vi "ble_read_write_characteristics.vi"() -> ()   [LabVIEW 2021]
uses:
  <vilib>/BLE/type_def/connection_status_bundle.ctl
  <vilib>/BLE/type_def/address_type.ctl
  <vilib>/BLE/ble_functions/ble_write_by_service_characteristic_uint8array.vi
  <vilib>/Utility/inputDevices.llb/mouseAcquire.vi
  <vilib>/Utility/inputDevices.llb/closeMouse.vi
panel:
  in  "Emergency Stop":bool
  out "Current Mouse Coordinates":T1
  out "Mouse Status":cluster{"Clicked?":bool}
  out "Drawing":cluster{i32[], i32[]}[](graph)
  in  "Clear Drawing":bool
  out "Connected":bool
  out "Device Name":string
  in  "Address Type":T2=1 items=["Public", "Random"]
  out "Handle table":string[][](array[string])
  out "Connection Status":T3={"MAC Address"="", "cnx handle"=0, "cnx flags"=0, "Address Type"=125, "Connection Interval (ms)"=125, "Timeout(ms)"=125, "Latency"=0, "bonding handle"=0} {"Address Type" items=["Public", "Random"]}
  out "Scanning":bool
  in  "Continue":bool
  in  "MAC Address":string
  in  "COM Bluegiga in":refnum<visa-resource-name>="COM5"
  out "Devices":string[][](array[string])
  out "BLED112 Dongle Info":string
  # "This VI an example of scanning for BLE devices using the \nBLED112 Bluetooth Smart Dongle by Bluegiga\nhttps://www.bluegiga.com/en-US/products/bled112-bluetooth-smart-dongle/\n\nand\nBLE (Bluetooth Low Energy) toolkit for LabVIEW\nww.\n\nInstructions:\nBefore running the VI\n1. Select the COM port for the BLED112 USB receiver\n(You can verify this in the Device Manager)\n\n2. Run the VI\n\n3. The VI will reset the dongle and scan for available BLE devices\n \n4. Introduce the MAC Address and Address Type of the device you want to connect and click in the CONTINUE button to connect with it\n\n5. The VI will read the Characteristic 0x2A00 of the Service 0x1800 which contains \nthe Device Name\n\nhttps://www.bluetooth.com/specifications/gatt/viewer?attributeXmlFile=org.bluetooth.service.generic_access.xml&u=org.bluetooth.service.generic_access.xml"
  # "SCAN"
  # "RSSI (power)"
  # "Advertising Package Type"
  # "MAC Address"
  # "Address Type"
  # "Friendly name"
  # "DEVICES FOUND"
  # "Introduce the MAC Address and Address Type of the device you want to connect and click in the CONTINUE button"
  # "CONNECT"
  # "READING DEVICE NAME"
  # "Service 0x1800\nCharacteristic 0x2A00\nDevice Name"
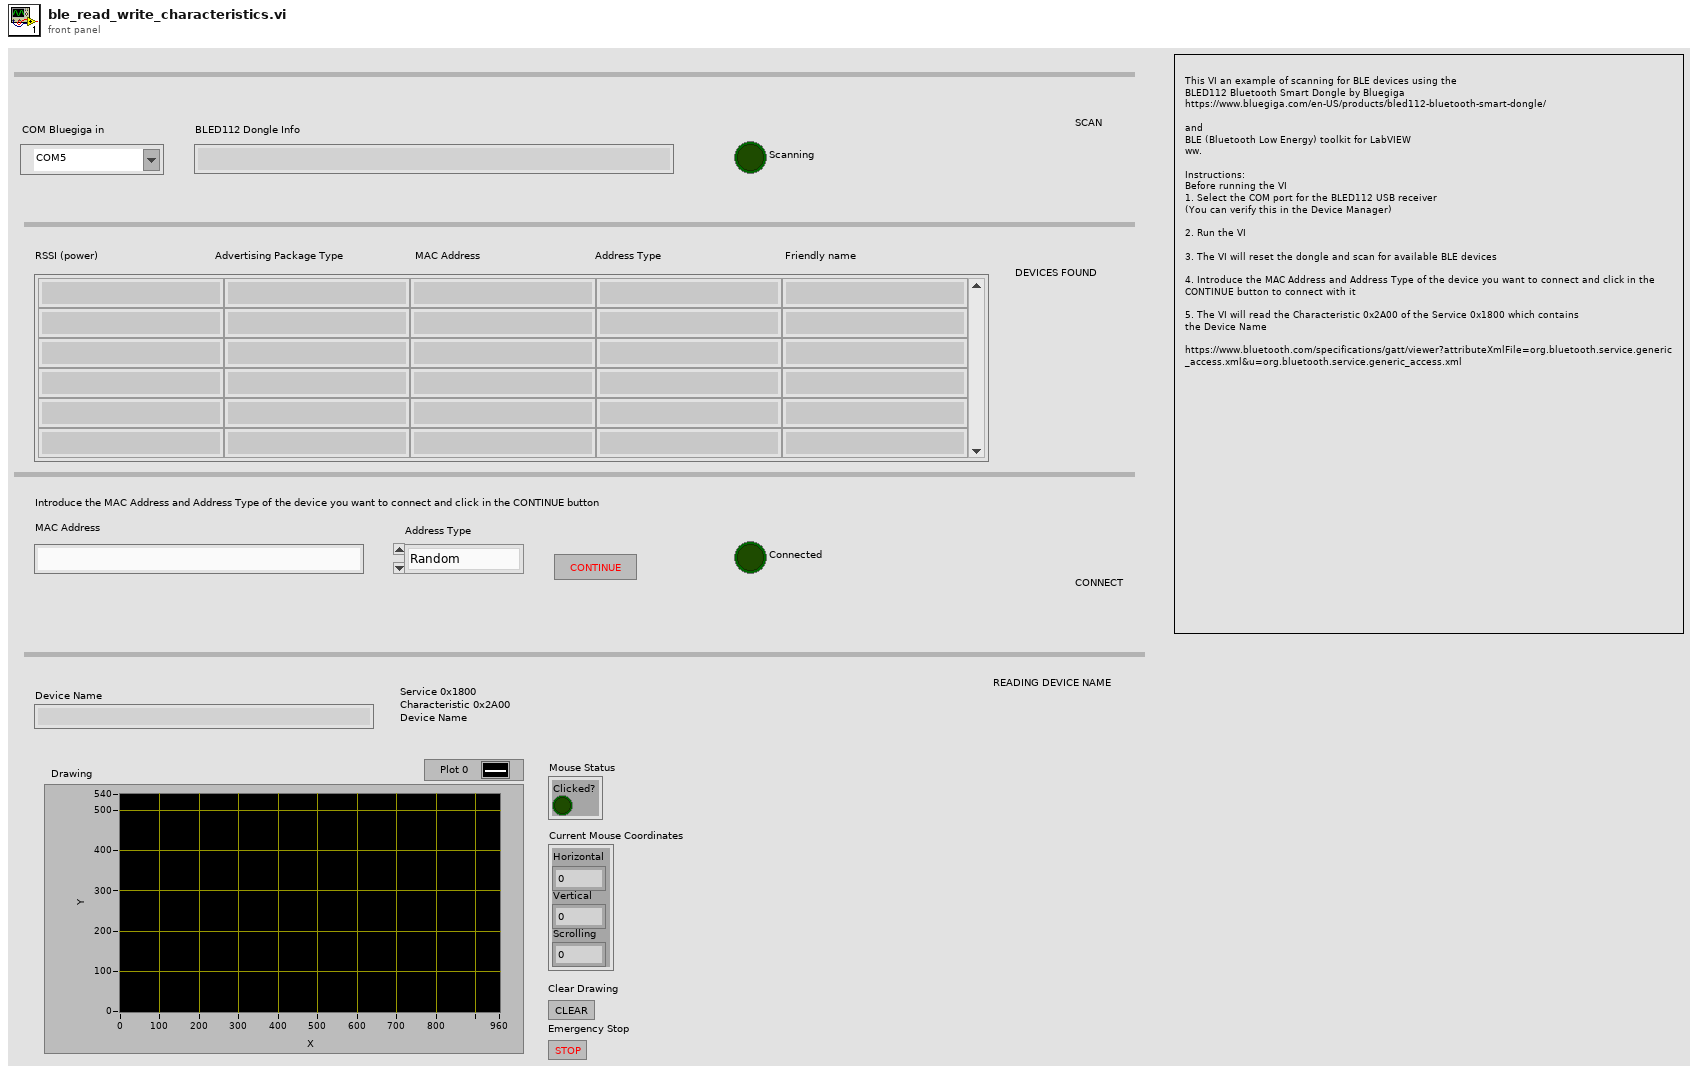
[diagram p1: front panel]
types:
  T1 = cluster{"Horizontal":i32, "Vertical":i32, "Scrolling":i32}
  T2 = typedef "address_type.ctl" = u8
  T3 = typedef "connection_status_bundle.ctl" = cluster{"MAC Address":string, "cnx handle":u8, "cnx flags":u8, "Address Type":T2, "Connection Interval (ms)":u16, "Timeout(ms)":u16, "Latency":u16, "bonding handle":u8}
  T4 = cluster{"Horizontal Array":i32[], "Vertical Array":i32[]}
  T5 = cluster{"Horizontal Array":i32[], "Vertical Array":i32[]}[]
  T6 = cluster{"button 1":bool, "button 2":bool, "button 3":bool, "button 4":bool}
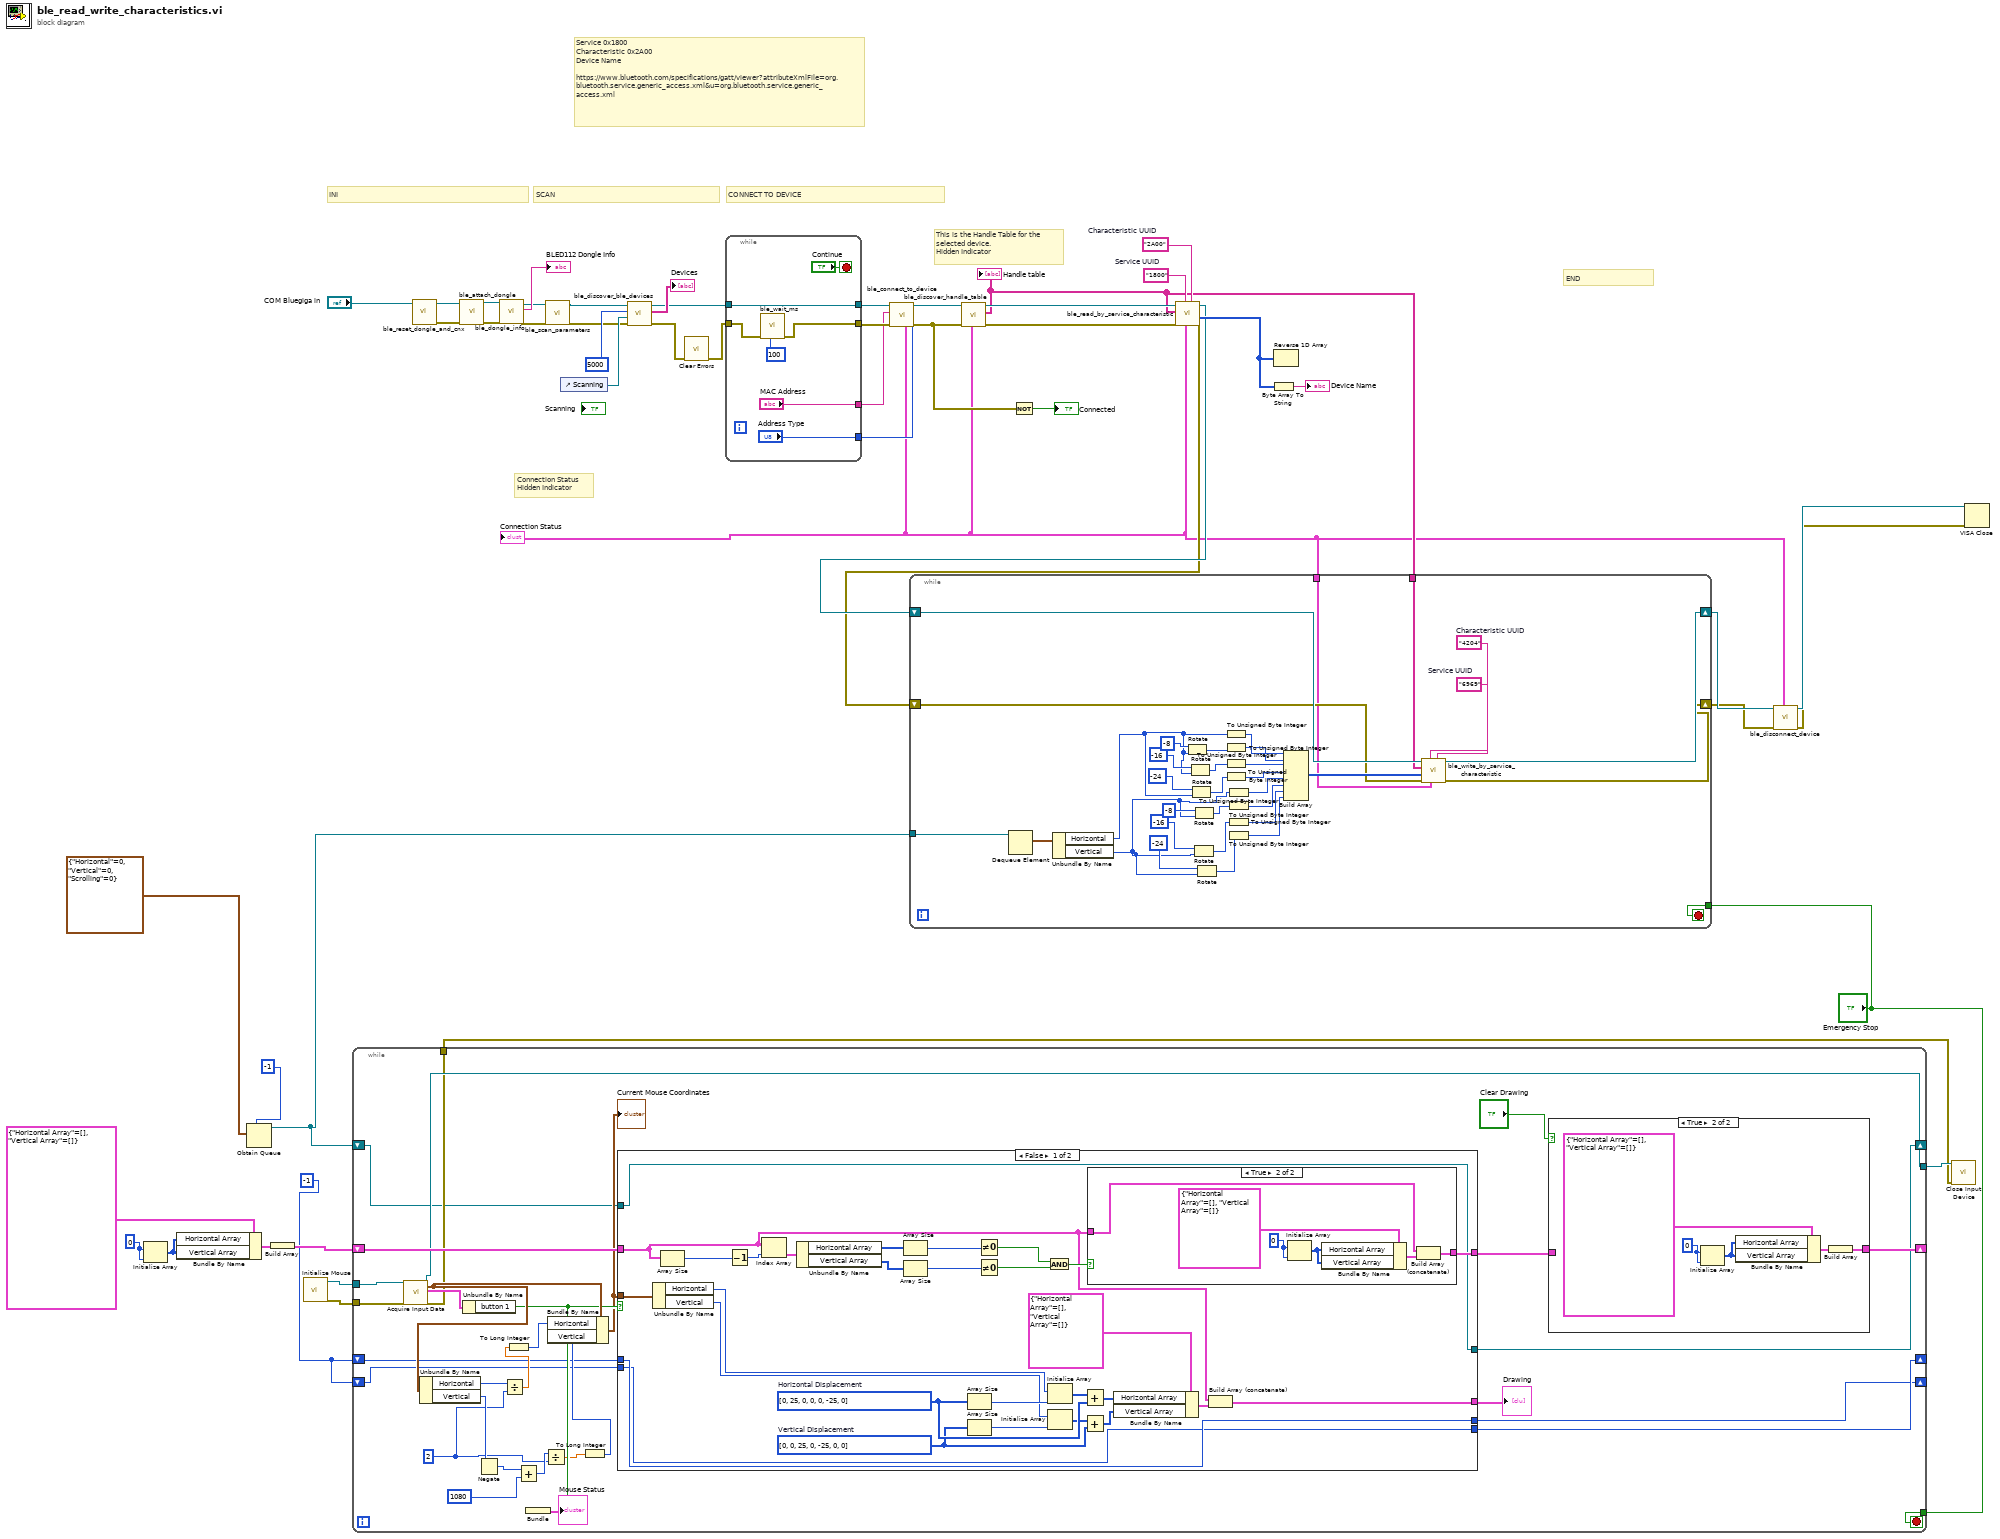
[diagram p0: block diagram]
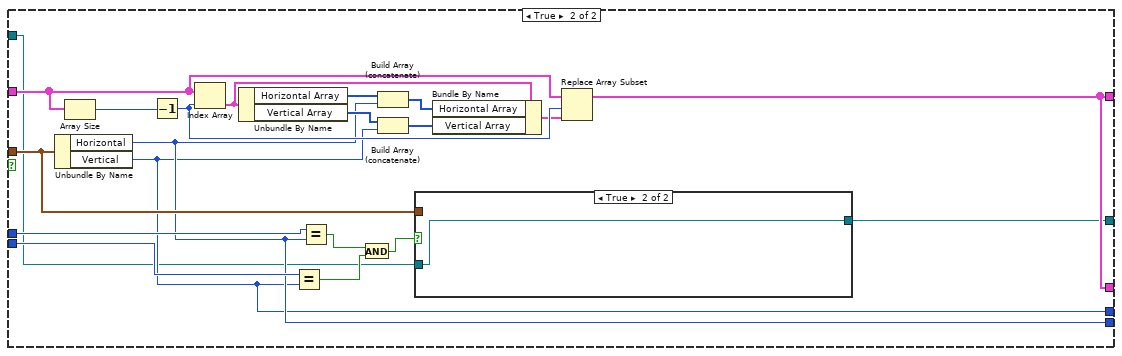
[diagram p4: hidden frame]
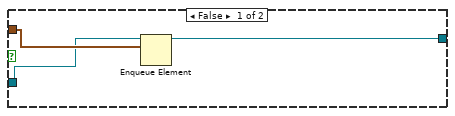
[diagram p5: hidden frame]
diagram:
  w10 = -1
  w16 = 0
  w21 = "2A00"  # Characteristic UUID
  w23 = "1800"  # Service UUID
  # "Connection Status\nHidden Indicator"
  # "Service 0x1800\nCharacteristic 0x2A00\nDevice Name\n\nhttps://www.bluetooth.com/specifications/gatt/viewer?attributeXmlFile=org.bluetooth.service.generic_access.xml&u=org.bluetooth.service.generic_access.xml"
  # "This is the Handle Table for the\nselected device. \nHidden Indicator"
  # "CONNECT TO DEVICE"
  # "SCAN"
  # "END"
  # "INI"
  n1 = Initialize Array(w16, w16) -> (w14:i32[])
  n2 = Bundle By Name(cluster=T4 {"Horizontal Array"=[], "Vertical Array"=[]}, "Horizontal Array"=w14, "Vertical Array"=w14) -> (w17:T4)
  n3 = Obtain Queue(max queue size (-1, unlimited)=-1, element data type=T1 {"Horizontal"=0, "Vertical"=0, "Scrolling"=0}) -> (queue out=w8:refnum<queue>)  [unwired: 3 in, 2 out]
  n4 = Build Array(w17) -> (w15:T5)
  n5 = call <vilib>:"Initialize Mouse.vi"() -> ("error out"=w19:errorcluster, "device ID"=w20:refnum<k1>)  [unwired: 10 in]
  n6 = while {
    tunnel: w20 -> [w82]
    tunnel: w19 -> [w81]
    shift-right: [w71] -> _
    shift-left: w15 -> [w75]
    tunnel: [w70] -> w13
    tunnel: [w69] -> w12
    shift-right: [w56] -> _
    shift-left: w10 -> [w59]
    shift-right: [w55] -> _
    shift-left: w10 -> [w58]
    shift-right: [w53] -> _
    shift-left: w8 -> [w54]
    tunnel: "Emergency Stop" -> [w52]
    stop <- w52 stop-if-true
    w62 = 2
    n7 = call-poly <vilib>:"Acquire Input Data.vi"("device ID"=w82, "error in (no error)"=w81) -> ("device ID"=w70:refnum<k1>, "axis info"=w79:T1, "button info"=w80:T6, "error out"=w69:errorcluster)  [unwired: 14 in]
    n8 = Unbundle By Name(w79) -> ("Horizontal"=w63:i32, "Vertical"=w78:i32)
    n9 = Unbundle By Name(w80) -> ("button 1"=w76:bool)
    n10 = Negate(x=w78) -> (-x=w68:i32)
    n11 = Divide(x=w63, y=w62) -> (x/y=w60:dbl)
    n12 = To Long Integer(number=w60) -> (32bit integer=w61:i32)
    n13 = Add(x=w68, y=1080) -> (x+y=w66:i32)
    n14 = Bundle("button 1"=w76) -> (→"Mouse Status":cluster{"button 1":bool})  [unwired: 1 in]
    n15 = Divide(x=w66, y=w62) -> (x/y=w65:dbl)
    n16 = To Long Integer(number=w65) -> (32bit integer=w64:i32)
    n17 = Bundle By Name(cluster=w79, "Horizontal"=w61, "Vertical"=w64) -> (w57:T1)
    "Current Mouse Coordinates" <- w57
    n18 = case shown="False" w76 {
      tunnel: w75 -> [w104 w138]
      tunnel: w57 -> [w106 w129]
      tunnel: [w107 w135] -> w72
      tunnel: [w102 w135] -> w74
      tunnel: w59 -> [w91 w131]
      tunnel: w58 -> [w90 w130]
      tunnel: [w90 w128] -> w56
      tunnel: [w91 w127] -> w55
      tunnel: w54 -> [w89 w126]
      tunnel: [w89 w125] -> w53
      frame False {
        w94 = i32[] [0, 0, 25, 0, -25, 0, 0]  # Vertical Displacement
        w96 = i32[] [0, 25, 0, 0, 0, -25, 0]  # Horizontal Displacement
        n19 = Unbundle By Name(w106) -> ("Horizontal"=w101:i32, "Vertical"=w99:i32)
        n20 = Array Size(array=w104) -> (size(s)=w115:i32)
        n21 = Decrement(x=w115) -> (x-1=w117:i32)
        n22 = Index Array(array=w104, index=w117) -> (element=w116:T4)
        n23 = Unbundle By Name(w116) -> ("Horizontal Array"=w114:i32[], "Vertical Array"=w113:i32[])
        n24 = Array Size(array=w114) -> (size(s)=w112:i32)
        n25 = Array Size(array=w113) -> (size(s)=w111:i32)
        n26 = Array Size(array=w96) -> (size(s)=w100:i32)
        n27 = Array Size(array=w94) -> (size(s)=w98:i32)
        n28 = Not Equal To 0?(x=w112) -> (x != 0?=w110:bool)
        n29 = Not Equal To 0?(x=w111) -> (x != 0?=w109:bool)
        n30 = And(x=w110, y=w109) -> (x .and. y?=w108:bool)
        n31 = Initialize Array(w101, w100) -> (w97:i32[])
        n32 = Initialize Array(w99, w98) -> (w95:i32[])
        n33 = Add(x=w97, y=w96) -> (x+y=w92:i32[])
        n34 = Add(x=w95, y=w94) -> (x+y=w93:i32[])
        n35 = case shown="True" w108 {
          tunnel: w104 -> [w118 w122]
          tunnel: [w118 w119] -> w107
          frame False {
          }
          frame True {
            w123 = 0
            n36 = Initialize Array(w123, w123) -> (w124:i32[])
            n37 = Bundle By Name(cluster=T4 {"Horizontal Array"=[], "Vertical Array"=[]}, "Horizontal Array"=w124, "Vertical Array"=w124) -> (w120:T4)
            n38 = Build Array (concatenate)(w122, w120) -> (w119:T5)
          }
        }
        n39 = Bundle By Name(cluster=T4 {"Horizontal Array"=[], "Vertical Array"=[]}, "Horizontal Array"=w92, "Vertical Array"=w93) -> (w103:T4)
        n40 = Build Array (concatenate)(w104, w103) -> (w102:T5)
      }
      frame True {
        n41 = Unbundle By Name(w129) -> ("Horizontal"=w128:i32, "Vertical"=w127:i32)
        n42 = Array Size(array=w138) -> (size(s)=w144:i32)
        n43 = Decrement(x=w144) -> (x-1=w137:i32)
        n44 = Index Array(array=w138, index=w137) -> (element=w141:T4)
        n45 = Unbundle By Name(w141) -> ("Horizontal Array"=w143:i32[], "Vertical Array"=w142:i32[])
        n46 = Equal?(x=w130, y=w127) -> (x = y?=w133:bool)
        n47 = Equal?(x=w131, y=w128) -> (x = y?=w134:bool)
        n48 = And(x=w134, y=w133) -> (x .and. y?=w132:bool)
        n49 = Build Array (concatenate)(w143, w128) -> (w140:i32[])
        n50 = Build Array (concatenate)(w142, w127) -> (w139:i32[])
        n51 = case shown="True" w132 {
          tunnel: w129 -> [w147 _]
          tunnel: w126 -> [w146 w148]
          tunnel: [w145 w148] -> w125
          frame False {
            n52 = Enqueue Element(queue=w146, element=w147) -> (queue out=w145:refnum<queue>)  [unwired: 2 in, 2 out]
          }
          frame True {
          }
        }
        n53 = Bundle By Name(cluster=w141, "Horizontal Array"=w140, "Vertical Array"=w139) -> (w136:T4)
        n54 = Replace Array Subset(array=w138, new element=w136, index=w137) -> (w135:T5)
      }
    }
    "Drawing" <- w74
    n55 = case shown="True" "Clear Drawing" {
      tunnel: w72 -> [w83 _]
      tunnel: [w83 w84] -> w71
      frame False {
      }
      frame True {
        w86 = 0
        n56 = Initialize Array(w86, w86) -> (w88:i32[])
        n57 = Bundle By Name(cluster=T4 {"Horizontal Array"=[], "Vertical Array"=[]}, "Horizontal Array"=w88, "Vertical Array"=w88) -> (w87:T4)
        n58 = Build Array(w87) -> (w84:T5)
      }
    }
  }
  n59 = call <vilib>:"ble_reset_dongle_and_cnx.vi"("COM Bluegiga in"="COM Bluegiga in") -> ("error out"=w35:errorcluster, "COM Bluegiga out"=w33:refnum<visa-resource-name>)  [unwired: 9 in]
  n60 = call <vilib>:"ble_attach_dongle.vi"("error in (no error)"=w35, "COM Bluegiga in"=w33) -> ("error out"=w37:errorcluster, "COM Bluegiga out"=w36:refnum<visa-resource-name>)  [unwired: 8 in]
  n61 = call <vilib>:"ble_dongle_info.vi"("error in (no error)"=w37, "COM Bluegiga in"=w36) -> ("error out"=w43:errorcluster, "info"=→"BLED112 Dongle Info":string, "COM Bluegiga out"=w44:refnum<visa-resource-name>)  [unwired: 7 in]
  n62 = call <vilib>:"ble_scan_parameters.vi"("error in (no error)"=w43, "COM Bluegiga in"=w44) -> ("error out"=w41:errorcluster, "COM Bluegiga out"=w42:refnum<visa-resource-name>)  [unwired: 7 in, 1 out]
  n63 = control-ref of="Scanning"() -> (w47:refnum<vi>)
  n64 = call <vilib>:"ble_discover_ble_devices.vi"("error in (no error)"=w41, "LED ref"=w47, "Scan Duration (10000ms)"=u32 5000, "COM Bluegiga in"=w42) -> ("error out"=w31:errorcluster, "Devices"=→"Devices":string[][], "COM Bluegiga out"=w48:refnum<visa-resource-name>)  [unwired: 5 in]
  n65 = call <vilib>:"Clear Errors.vi"("error in (no error)"=w31) -> ("error out"=w30:errorcluster)  [unwired: 5 in, 1 out]
  n66 = while {
    tunnel: w30 -> [w154]
    tunnel: [w153] -> w46
    tunnel: w48 -> [w153]
    tunnel: [w152] -> w45
    tunnel: ["MAC Address"] -> w38
    tunnel: ["Address Type"] -> w29
    stop <- "Continue" stop-if-true
    n67 = call <vilib>:"ble_wait_ms.vi"("milliseconds to wait (100)"=u32 100, "error in (no error)"=w154) -> ("error out"=w152:errorcluster)  [unwired: 9 in]
  }
  n68 = call <vilib>:"ble_connect_to_device.vi"("Address Type"=w29, "error in (no error)"=w45, "MAC Address"=w38, "COM Bluegiga in"=w46) -> ("error out"=w24:errorcluster, "COM Bluegiga out"=w32:refnum<visa-resource-name>, "Connection Status"=w3:T3)  [unwired: 5 in]
  "Connection Status" <- w3
  n69 = call <vilib>:"ble_discover_handle_table.vi"("Connection Status"=w3, "error in (no error)"=w24, "COM Bluegiga in"=w32) -> ("error out"=w28:errorcluster, "Handle table"=w4:string[][], "COM Bluegiga out"=w27:refnum<visa-resource-name>)  [unwired: 6 in]
  "Handle table" <- w4
  n70 = Not(x=w24) -> (.not. x?=→"Connected":bool)
  n71 = call <vilib>:"ble_read_by_service_characteristic.vi"("Characteristic UUID"=w21, "Connection Status"=w3, "Service UUID"=w23, "error in (no error)"=w28, "Handle table"=w4, "COM Bluegiga in"=w27) -> ("error out"=w5:errorcluster, "attribute value"=w22:u8[], "COM Bluegiga out"=w6:refnum<visa-resource-name>)  [unwired: 2 in, 1 out]
  n72 = while {
    tunnel: "Emergency Stop" -> [w189]
    tunnel: w8 -> [w188]
    shift-right: [w163] -> w2
    shift-left: w6 -> [w164]
    shift-right: [w161] -> w1
    shift-left: w5 -> [w162]
    tunnel: w4 -> [w158]
    tunnel: w3 -> [w157]
    stop <- w189 stop-if-true
    w160 = "4204"  # Characteristic UUID
    w159 = "6969"  # Service UUID
    n73 = Dequeue Element(queue=w188) -> (element=w187:T1)  [unwired: 2 in, 3 out]
    n74 = Unbundle By Name(w187) -> ("Horizontal"=w166:i32, "Vertical"=w156:i32)
    n75 = Rotate(1:w166, 2:-8) -> (0:w178:i32)
    n76 = Rotate(1:w166, 2:-16) -> (0:w177:i32)
    n77 = Rotate(1:w166, 2:-24) -> (0:w176:i32)
    n78 = Rotate(1:w156, 2:-16) -> (0:w174:i32)
    n79 = Rotate(1:w156, 2:-8) -> (0:w175:i32)
    n80 = Rotate(1:w156, 2:-24) -> (0:w173:i32)
    n81 = To Unsigned Byte Integer(number=w166) -> (unsigned 8bit integer=w186:u8)
    n82 = To Unsigned Byte Integer(number=w178) -> (unsigned 8bit integer=w185:u8)
    n83 = To Unsigned Byte Integer(number=w177) -> (unsigned 8bit integer=w184:u8)
    n84 = To Unsigned Byte Integer(number=w176) -> (unsigned 8bit integer=w183:u8)
    n85 = To Unsigned Byte Integer(number=w156) -> (unsigned 8bit integer=w182:u8)
    n86 = To Unsigned Byte Integer(number=w175) -> (unsigned 8bit integer=w181:u8)
    n87 = To Unsigned Byte Integer(number=w174) -> (unsigned 8bit integer=w180:u8)
    n88 = To Unsigned Byte Integer(number=w173) -> (unsigned 8bit integer=w179:u8)
    n89 = Build Array(w186, w185, w184, w183, w182, w181, w180, w179) -> (w165:u8[])
    n90 = call-poly <vilib>:"ble_write_by_service_characteristic.vi"("Characteristic UUID"=w160, "Connection Status"=w157, "Service UUID"=w159, "error in (no error)"=w162, "data"=w165, "Handle table"=w158, "COM Bluegiga in"=w164) -> ("error out"=w161:errorcluster, "COM Bluegiga out"=w163:refnum<visa-resource-name>)  [unwired: 3 in]
  }
  n91 = Byte Array To String(unsigned byte array=w22) -> (string=→"Device Name":string)
  n92 = Reverse 1D Array(array=w22) -> ()  [unwired: 1 out]
  n93 = call <vilib>:"ble_disconnect_device.vi"("Connection Status"=w3, "error in (no error)"=w1, "COM Bluegiga in"=w2) -> ("error out"=w39:errorcluster, "COM Bluegiga out"=w40:refnum<visa-resource-name>)  [unwired: 7 in]
  n94 = call-poly <vilib>:"Close Input Device.vi"("error in (no error)"=w12, "device ID"=w13) -> ()  [unwired: 8 in, 1 out]
  n95 = VISA Close(VISA resource name=w40, error in (no error)=w39) -> ()  [unwired: 1 out]
